vi "getsnjob.vi"(4 "sample port":refnum<visa-resource-name>[](array[refnum])) -> (0 "sample sn":string[](array[string]))   [LabVIEW 2012]
uses:
  globalstatus.vi
  globalreport.vi
panel:
  out "error":errorcluster[](array[cluster])
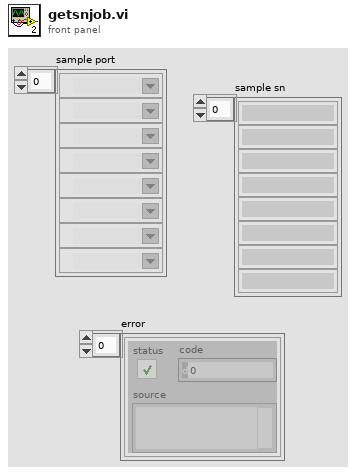
[diagram p1: front panel]
types:
  T1 = cluster{"PORT":string, "SN":string, "DO 0":string, "DO 1":string, "DO 2":string, "DO 3":string, "DO 4":string, "DO 5":string, "DO 6":string, "result":string, "error":string}[]
  T2 = cluster{"PORT":string, "SN":string, "RED DAC":dbl, "BLUE DAC":dbl, "RED AMP":dbl, "BLUE AMP":dbl, "T0":dbl, "T1":dbl, "T2":dbl, "T3":dbl, "T4":dbl, "T5":dbl, "T6":dbl, "A0":dbl, "A1":dbl, "A2":dbl, "A3":dbl, "B0":dbl, "B1":dbl, "B2":dbl, "C1":dbl, "C0":dbl, "result":string, "error":string}[]
  T3 = cluster{"PORT":string, string, "RED DAC":dbl, "BLUE DAC":dbl, "RED AMP":dbl, "BLUE AMP":dbl, "T0":dbl, "T1":dbl, "T2":dbl, "T3":dbl, "T4":dbl, "T5":dbl, "T6":dbl, "A0":dbl, "A1":dbl, "A2":dbl, "A3":dbl, "B0":dbl, "B1":dbl, "B2":dbl, "C1":dbl, "C0":dbl, string, string}
  T4 = cluster{"PORT":string, "String":string, "RED DAC":dbl, "BLUE DAC":dbl, "RED AMP":dbl, "BLUE AMP":dbl, "T0":dbl, "T1":dbl, "T2":dbl, "T3":dbl, "T4":dbl, "T5":dbl, "T6":dbl, "A0":dbl, "A1":dbl, "A2":dbl, "A3":dbl, "B0":dbl, "B1":dbl, "B2":dbl, "C1":dbl, "C0":dbl, string, string}
  T5 = cluster{"PORT":string, string, "DO 0":string, "DO 1":string, "DO 2":string, "DO 3":string, "DO 4":string, "DO 5":string, "DO 6":string, string, string}
  T6 = cluster{"PORT":string, "String":string, "DO 0":string, "DO 1":string, "DO 2":string, "DO 3":string, "DO 4":string, "DO 5":string, "DO 6":string, "result":string, "error":string}
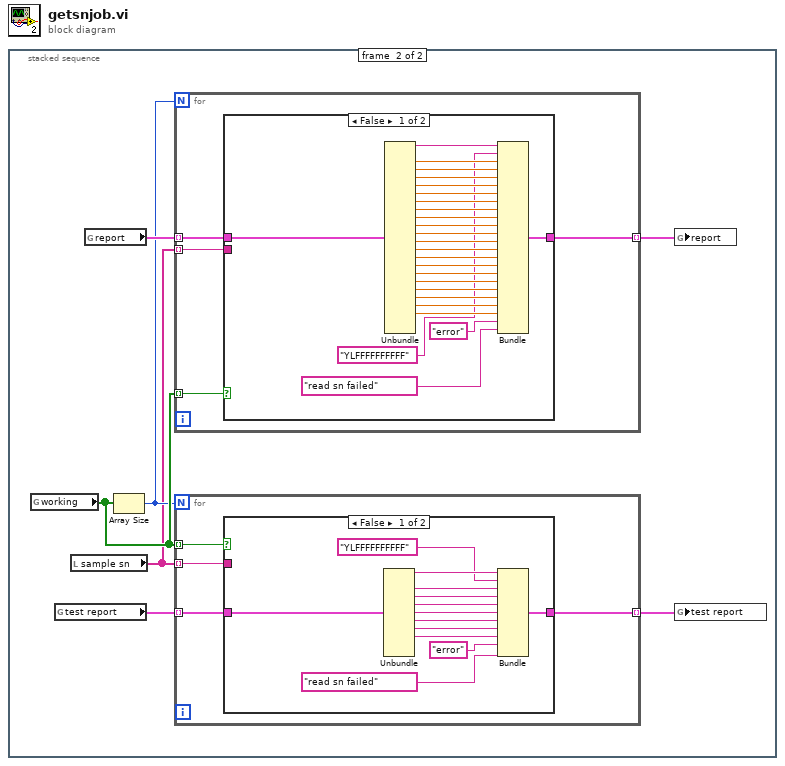
[diagram p0: block diagram]
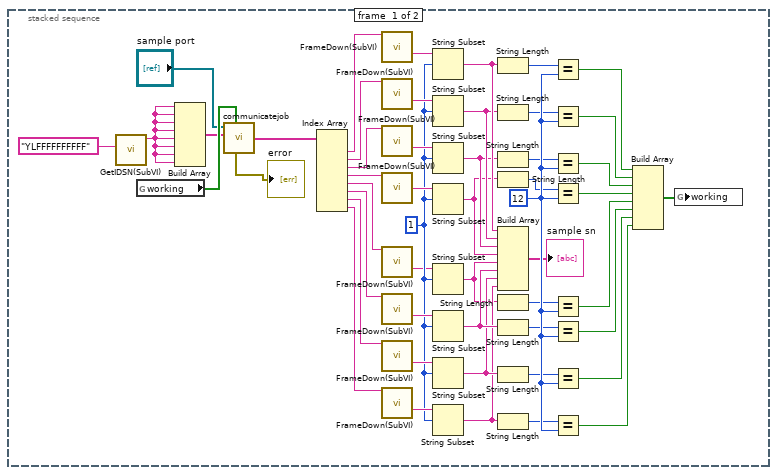
[diagram p2: hidden frame]
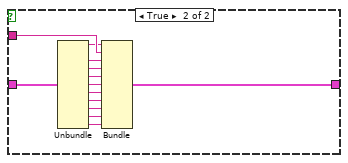
[diagram p3: hidden frame]
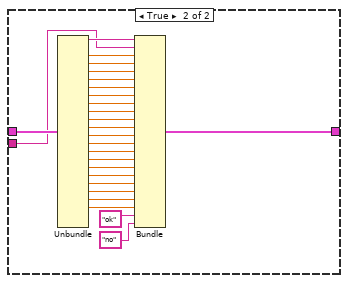
[diagram p4: hidden frame]
diagram:
  n1 = stacked-sequence {
    frame #0 {
      w5 = 1
      w51 = 12
      n2 = call "GetIDSN(SubVI).vi"("sn"="YLFFFFFFFFFF") -> ("output frame"=w21:string)  [unwired: 10 in]
      n3 = global read "globalstatus.vi" "working"() -> (w25:bool[])
      n4 = Build Array(w21, w21, w21, w21, w21, w21, w21, w21) -> (w24:string[])
      n5 = call "communicatejob.vi"("sample port"="sample port", "condition"=w25, "send command"=w24) -> ("error"=→"error":errorcluster[], "receive command"=w26:string[])  [unwired: 2 in, 2 out]
      n6 = Index Array(array=w26) -> (element #1=w27:string, element #2=w28:string, element #3=w29:string, element #4=w30:string, element #5=w31:string, element #6=w32:string, element #7=w33:string, element #8=w34:string)  [unwired: 8 in]
      n7 = call "FrameDown(SubVI).vi"("input frame"=w27) -> ("data"=w20:string)  [unwired: 4 in, 10 out]
      n8 = call "FrameDown(SubVI).vi"("input frame"=w28) -> ("data"=w11:string)  [unwired: 4 in, 10 out]
      n9 = call "FrameDown(SubVI).vi"("input frame"=w29) -> ("data"=w7:string)  [unwired: 4 in, 10 out]
      n10 = call "FrameDown(SubVI).vi"("input frame"=w30) -> ("ob"=w8:string)  [unwired: 4 in, 10 out]
      n11 = call "FrameDown(SubVI).vi"("input frame"=w31) -> ("data"=w4:string)  [unwired: 4 in, 10 out]
      n12 = call "FrameDown(SubVI).vi"("input frame"=w32) -> ("data"=w18:string)  [unwired: 4 in, 10 out]
      n13 = call "FrameDown(SubVI).vi"("input frame"=w33) -> ("data"=w16:string)  [unwired: 4 in, 10 out]
      n14 = call "FrameDown(SubVI).vi"("input frame"=w34) -> ("data"=w14:string)  [unwired: 4 in, 10 out]
      n15 = String Subset(string=w20, offset (0)=w5) -> (substring=w19:string)  [unwired: 1 in]
      n16 = String Subset(string=w11, offset (0)=w5) -> (substring=w12:string)  [unwired: 1 in]
      n17 = String Subset(string=w7, offset (0)=w5) -> (substring=w10:string)  [unwired: 1 in]
      n18 = String Subset(string=w8, offset (0)=w5) -> (substring=w9:string)  [unwired: 1 in]
      n19 = String Subset(string=w4, offset (0)=w5) -> (substring=w6:string)  [unwired: 1 in]
      n20 = String Subset(string=w18, offset (0)=w5) -> (substring=w17:string)  [unwired: 1 in]
      n21 = String Subset(string=w16, offset (0)=w5) -> (substring=w15:string)  [unwired: 1 in]
      n22 = String Subset(string=w14, offset (0)=w5) -> (substring=w13:string)  [unwired: 1 in]
      n23 = String Length(string=w19) -> (length=w50:i32)
      n24 = String Length(string=w12) -> (length=w49:i32)
      n25 = String Length(string=w10) -> (length=w48:i32)
      n26 = String Length(string=w9) -> (length=w47:i32)
      n27 = Build Array(w19, w12, w10, w9, w6, w17, w15, w13) -> (→"sample sn":string[])
      n28 = String Length(string=w6) -> (length=w46:i32)
      n29 = String Length(string=w17) -> (length=w45:i32)
      n30 = String Length(string=w15) -> (length=w44:i32)
      n31 = String Length(string=w13) -> (length=w43:i32)
      n32 = Equal?(x=w50, y=w51) -> (x = y?=w42:bool)
      n33 = Equal?(x=w49, y=w51) -> (x = y?=w41:bool)
      n34 = Equal?(x=w48, y=w51) -> (x = y?=w40:bool)
      n35 = Equal?(x=w47, y=w51) -> (x = y?=w39:bool)
      n36 = Equal?(x=w46, y=w51) -> (x = y?=w38:bool)
      n37 = Equal?(x=w45, y=w51) -> (x = y?=w37:bool)
      n38 = Equal?(x=w44, y=w51) -> (x = y?=w36:bool)
      n39 = Equal?(x=w43, y=w51) -> (x = y?=w35:bool)
      n40 = Build Array(w42, w41, w40, w39, w38, w37, w36, w35) -> (w1:bool[])
      n41 = global write "globalstatus.vi" "working"(w1) -> ()
    }
    frame #1 {
      n42 = global read "globalstatus.vi" "working"() -> (w56:bool[])
      n43 = global read "globalreport.vi" "test report"() -> (w54:T1)
      n44 = local read "sample sn"() -> (w52:string[])
      n45 = global read "globalreport.vi" "report"() -> (w58:T2)
      n46 = Array Size(array=w56) -> (size(s)=w55:i32)
      n47 = for {
        N: w55 -> [_]
        tunnel: w56 -> [w92] mode=indexing
        tunnel: w52 -> [w91] mode=indexing
        tunnel: w58 -> [w90] mode=indexing
        tunnel: [w89] -> w57 mode=indexing
        n48 = case shown="False" w92 {
          tunnel: w90 -> [w118 w144]
          tunnel: w91 -> [_ w121]
          tunnel: [w97 w123] -> w89
          frame False {
            n49 = Unbundle(w118) -> ("PORT"=w96:string, "RED DAC"=w98:dbl, "BLUE DAC"=w99:dbl, "RED AMP"=w100:dbl, "BLUE AMP"=w101:dbl, "T0"=w102:dbl, "T1"=w103:dbl, "T2"=w104:dbl, "T3"=w105:dbl, "T4"=w106:dbl, "T5"=w107:dbl, "T6"=w108:dbl, "A0"=w109:dbl, "A1"=w110:dbl, "A2"=w111:dbl, "A3"=w112:dbl, "B0"=w113:dbl, "B1"=w114:dbl, "B2"=w115:dbl, "C1"=w116:dbl, "C0"=w117:dbl)  [unwired: 3 out]
            n50 = Bundle("PORT"=w96, "YLFFFFFFFFFF", "RED DAC"=w98, "BLUE DAC"=w99, "RED AMP"=w100, "BLUE AMP"=w101, "T0"=w102, "T1"=w103, "T2"=w104, "T3"=w105, "T4"=w106, "T5"=w107, "T6"=w108, "A0"=w109, "A1"=w110, "A2"=w111, "A3"=w112, "B0"=w113, "B1"=w114, "B2"=w115, "C1"=w116, "C0"=w117, "error", "read sn failed") -> (w97:T3)  [unwired: 1 in]
          }
          frame True {
            n51 = Unbundle(w144) -> ("PORT"=w122:string, "RED DAC"=w143:dbl, "BLUE DAC"=w142:dbl, "RED AMP"=w141:dbl, "BLUE AMP"=w140:dbl, "T0"=w138:dbl, "T1"=w139:dbl, "T2"=w137:dbl, "T3"=w136:dbl, "T4"=w135:dbl, "T5"=w134:dbl, "T6"=w133:dbl, "A0"=w132:dbl, "A1"=w131:dbl, "A2"=w130:dbl, "A3"=w129:dbl, "B0"=w128:dbl, "B1"=w126:dbl, "B2"=w127:dbl, "C1"=w125:dbl, "C0"=w124:dbl)  [unwired: 3 out]
            n52 = Bundle("PORT"=w122, "String"=w121, "RED DAC"=w143, "BLUE DAC"=w142, "RED AMP"=w141, "BLUE AMP"=w140, "T0"=w138, "T1"=w139, "T2"=w137, "T3"=w136, "T4"=w135, "T5"=w134, "T6"=w133, "A0"=w132, "A1"=w131, "A2"=w130, "A3"=w129, "B0"=w128, "B1"=w126, "B2"=w127, "C1"=w125, "C0"=w124, "ok", "no") -> (w123:T4)  [unwired: 1 in]
          }
        }
      }
      n53 = for {
        N: w55 -> [_]
        tunnel: w56 -> [w62] mode=indexing
        tunnel: w54 -> [w61] mode=indexing
        tunnel: [w60] -> w53 mode=indexing
        tunnel: w52 -> [w59] mode=indexing
        n54 = case shown="False" w62 {
          tunnel: w61 -> [w75 w88]
          tunnel: [w74 w87] -> w60
          tunnel: w59 -> [_ w86]
          frame False {
            n55 = Unbundle(w75) -> ("PORT"=w73:string, "DO 0"=w71:string, "DO 1"=w70:string, "DO 2"=w69:string, "DO 3"=w68:string, "DO 4"=w67:string, "DO 5"=w66:string, "DO 6"=w65:string)  [unwired: 3 out]
            n56 = Bundle("PORT"=w73, "YLFFFFFFFFFF", "DO 0"=w71, "DO 1"=w70, "DO 2"=w69, "DO 3"=w68, "DO 4"=w67, "DO 5"=w66, "DO 6"=w65, "error", "read sn failed") -> (w74:T5)  [unwired: 1 in]
          }
          frame True {
            n57 = Unbundle(w88) -> ("PORT"=w85:string, "DO 0"=w84:string, "DO 1"=w83:string, "DO 2"=w82:string, "DO 3"=w81:string, "DO 4"=w80:string, "DO 5"=w79:string, "DO 6"=w78:string, "result"=w77:string, "error"=w76:string)  [unwired: 1 out]
            n58 = Bundle("PORT"=w85, "String"=w86, "DO 0"=w84, "DO 1"=w83, "DO 2"=w82, "DO 3"=w81, "DO 4"=w80, "DO 5"=w79, "DO 6"=w78, "result"=w77, "error"=w76) -> (w87:T6)  [unwired: 1 in]
          }
        }
      }
      n59 = global write "globalreport.vi" "report"(w57) -> ()
      n60 = global write "globalreport.vi" "test report"(w53) -> ()
    }
  }
